vi "dataset_info.vi"(9 "Analog Salita":dbl[][](array[numeric])) -> (1 "samples":i32, 2 "features":i32, 4 "size(s)":i32[](array[numeric]), 5 "samples_per_feature":i32)   [LabVIEW 2021, in "CALIBRATION.lvlib"]
uses:
  CALIBRATION.lvlib
panel:
  out "NaN found":bool
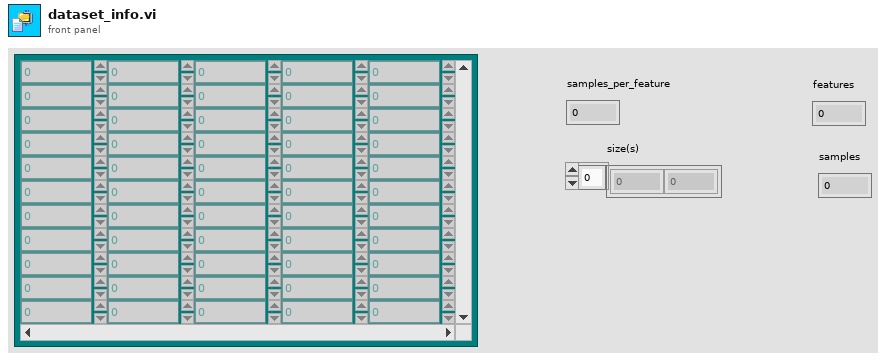
[diagram p1: front panel]
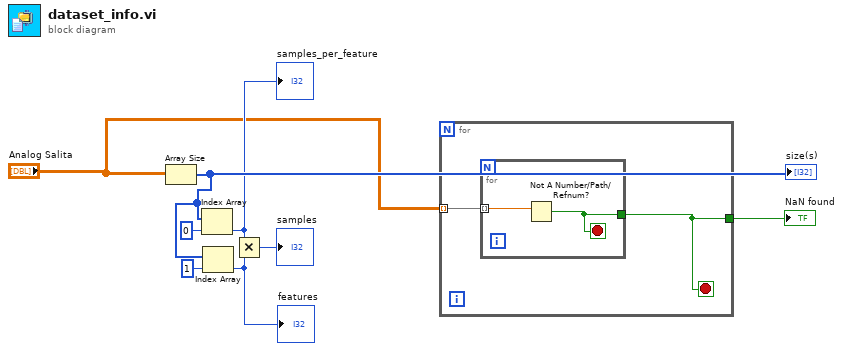
[diagram p0: block diagram]
diagram:
  n1 = Array Size(array="Analog Salita") -> (size(s)=w7:i32[])
  "size(s)" <- w7
  n2 = Index Array(array=w7, index=0) -> (element=w5:i32)
  "samples_per_feature" <- w5
  n3 = Index Array(array=w7, index=1) -> (element=w4:i32)
  "features" <- w4
  n4 = Multiply(x=w5, y=w4) -> (x*y=→"samples":i32)
  n5 = for {
    tunnel: "Analog Salita" -> [w10] mode=indexing
    tunnel: [w9] -> w1
    stop <- w9 stop-if-true
    n6 = for {
      tunnel: w10 -> [w12] mode=indexing
      tunnel: [w11] -> w9
      stop <- w11 stop-if-true
      n7 = Not A Number/Path/Refnum?(number/path/refnum=w12) -> (NaN/Path/Refnum?=w11:bool)
    }
  }
  "NaN found" <- w1
